vi "display_3s_stim_6s_ISI_12s_probes.vi"() -> ()   [LabVIEW 2019]
uses:
  <vilib>/Analysis/Matrix/Datatypes/RealMatrix.ctl
  <vilib>/Utility/file.llb/Write Delimited Spreadsheet (DBL).vi
  <vilib>/Analysis/Matrix/NI_Matrix.lvlib
panel:
  out "Num trials":u32=204
  out "ISI Time":dbl
  out "Stim TS":dbl
  out "Output":dbl[][](array[numeric])
  out "Output frame":T1
  out "Array temp1":T1
  out "Elapsed Time":dbl
  out "Display":bool=TRUE
  out "Trial":u32=1
  out "reward":dbl[](array[numeric])
  out "stim_id":dbl[](array[numeric])
  out "stim_loaded":dbl
  out "Timings":dbl[](array[numeric])
  out "Stimuli Loaded?":bool
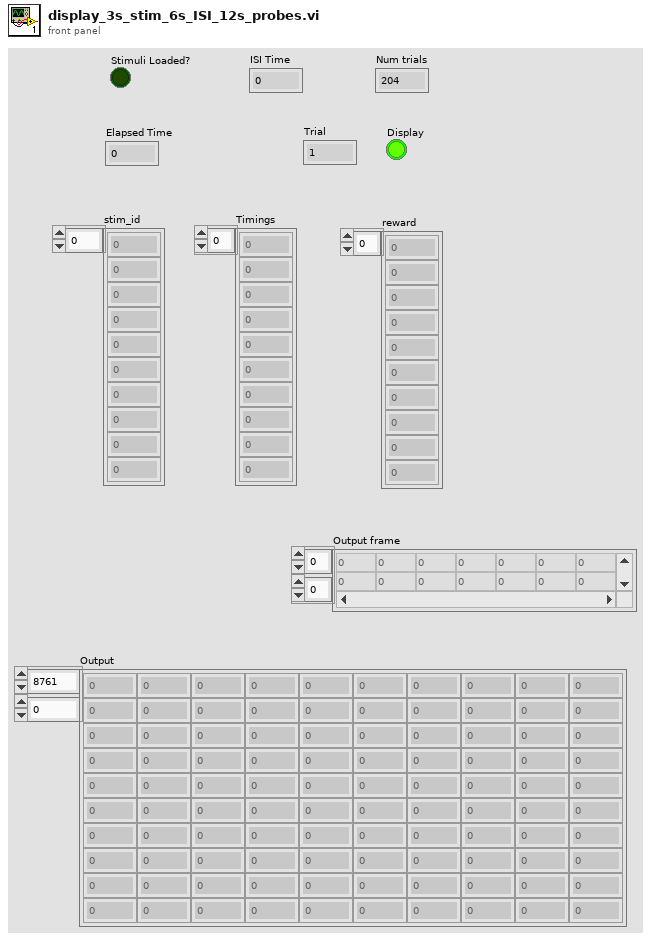
[diagram p1: front panel]
types:
  T1 = typedef "NI_Matrix.lvlib/RealMatrix.ctl" = dbl[][]
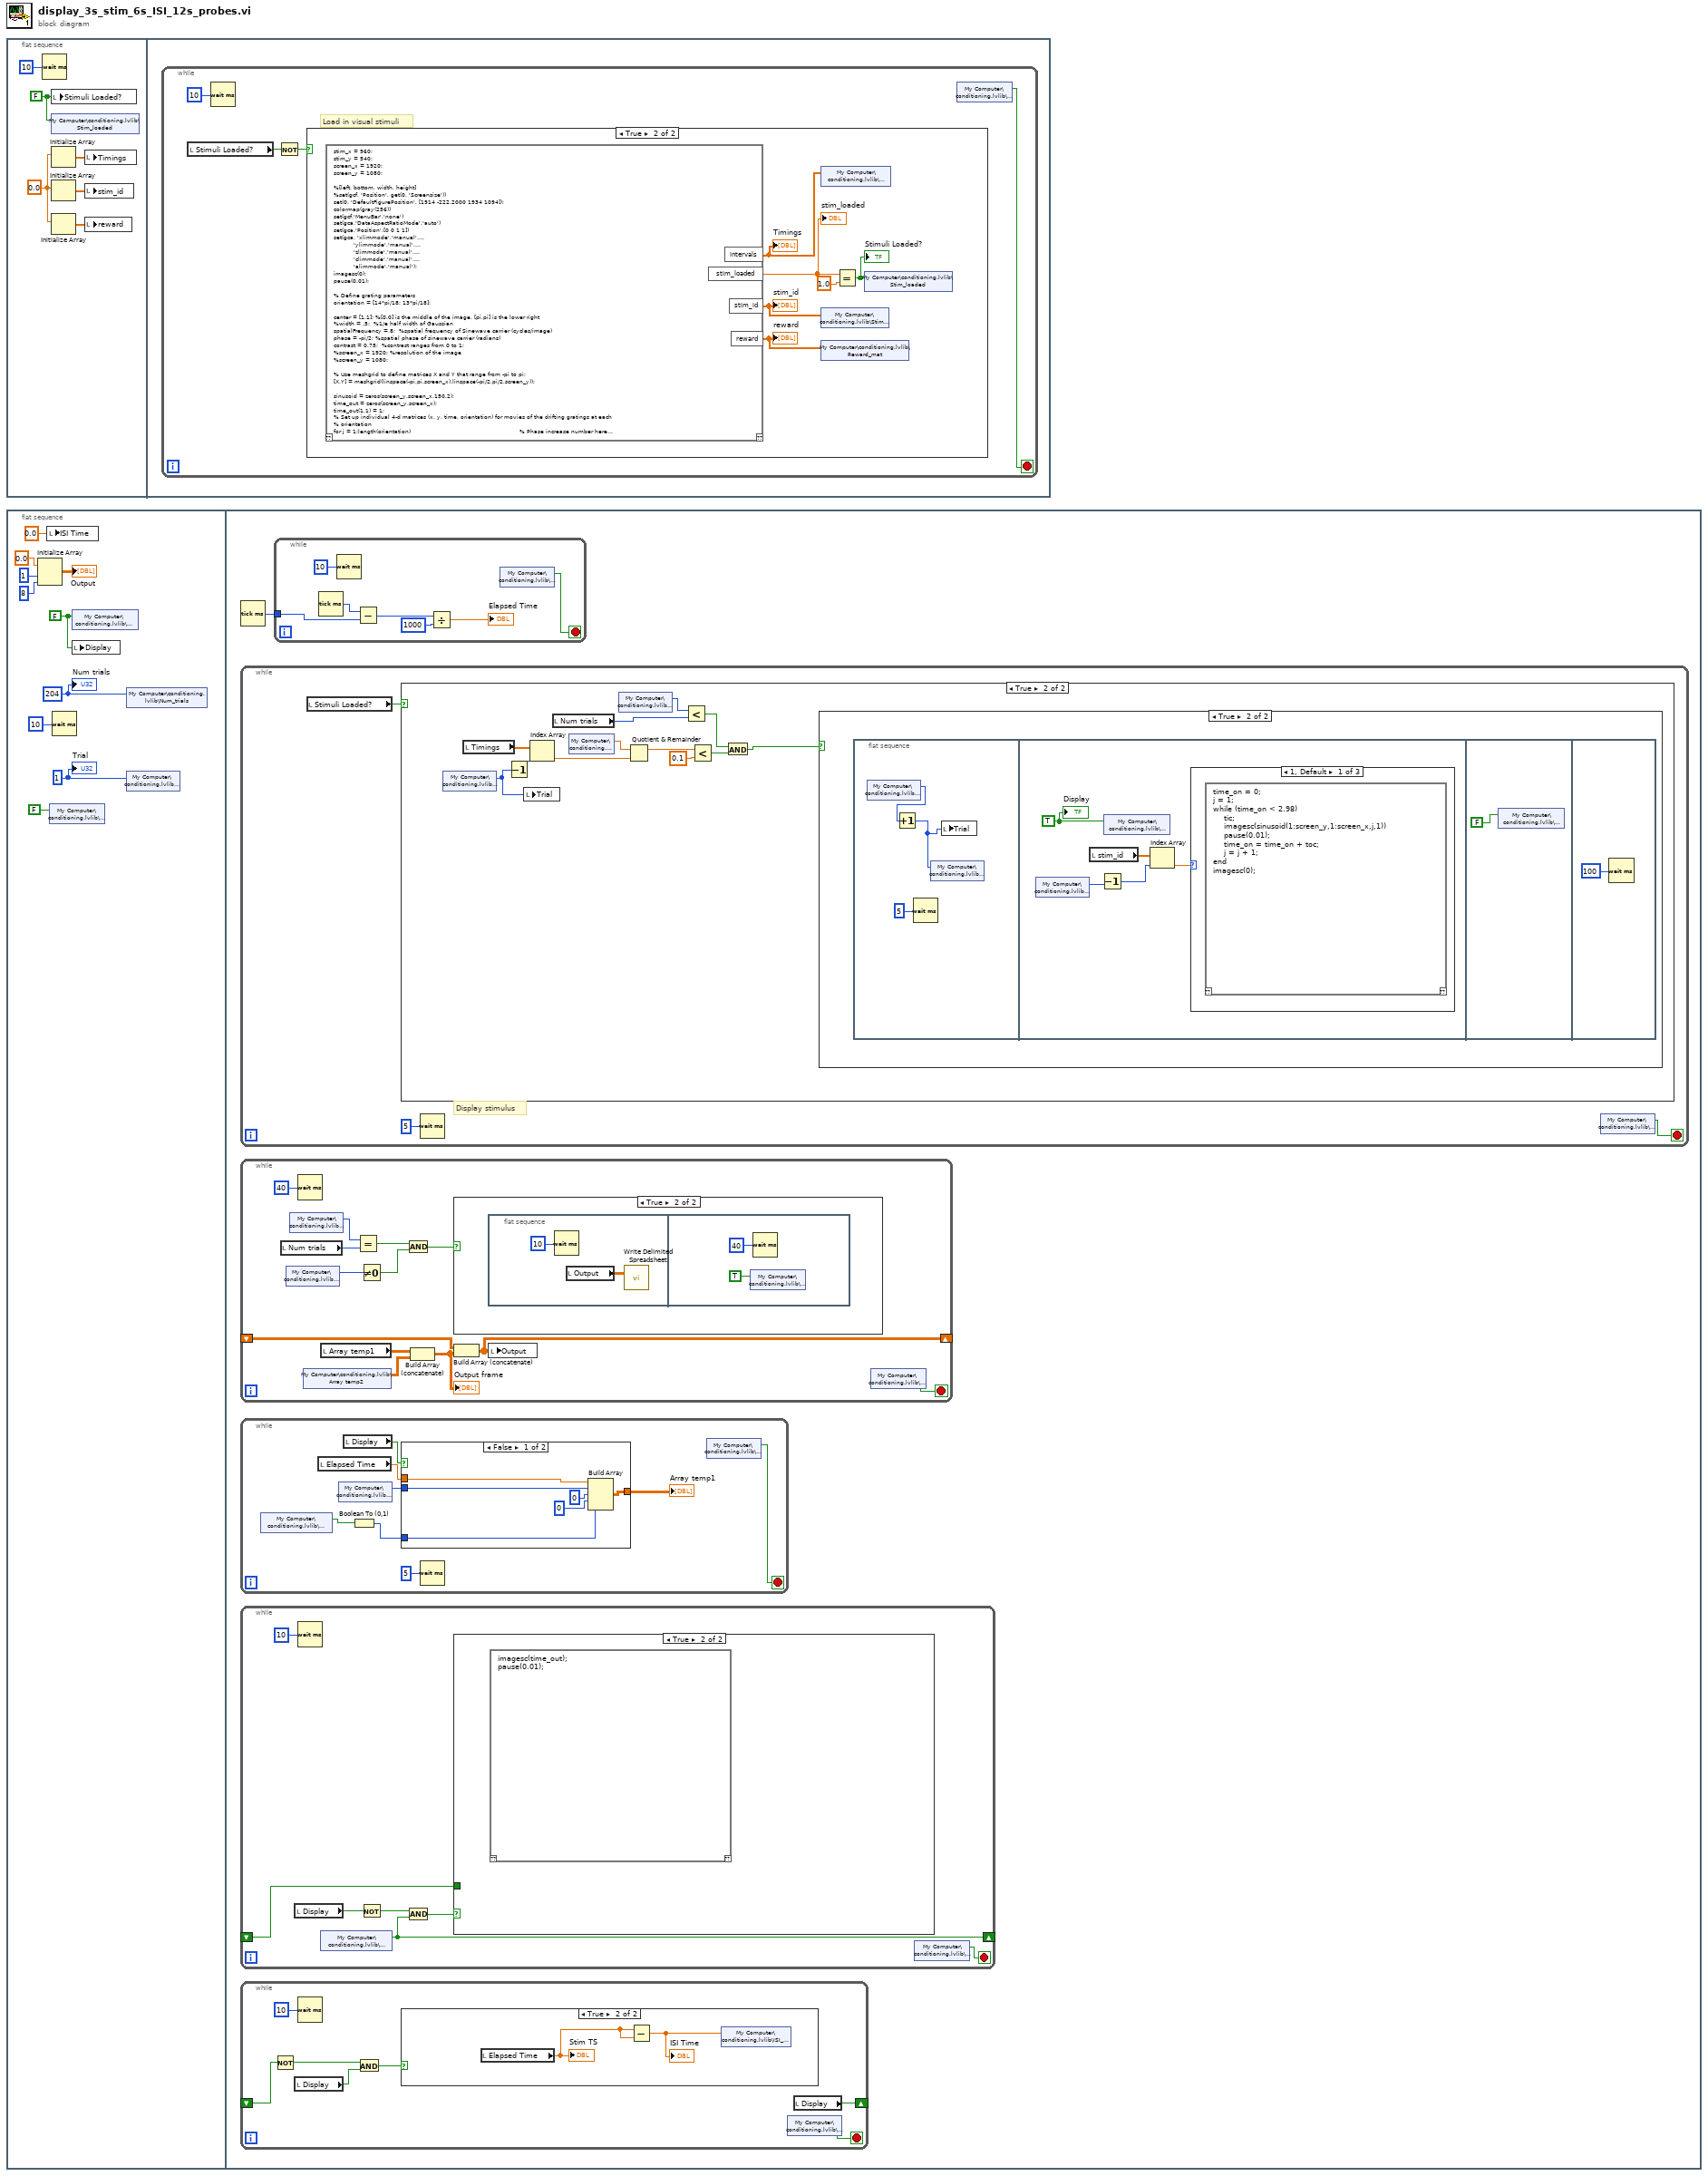
[diagram p0: block diagram]
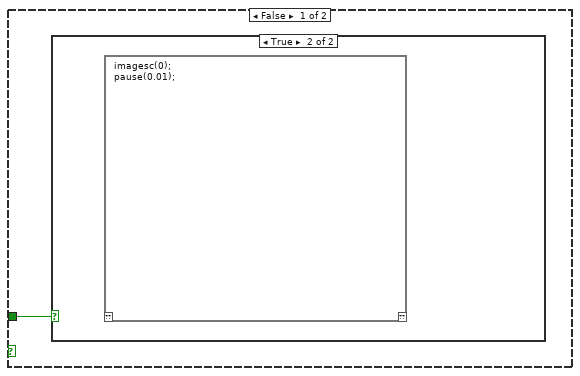
[diagram p3: hidden frame]
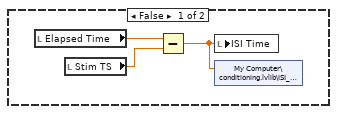
[diagram p5: hidden frame]
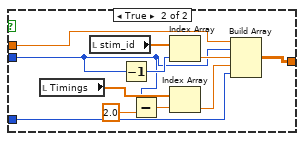
[diagram p6: hidden frame]
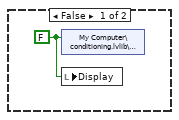
[diagram p9: hidden frame]
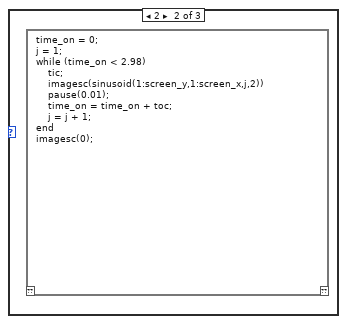
[diagram p10: hidden frame]
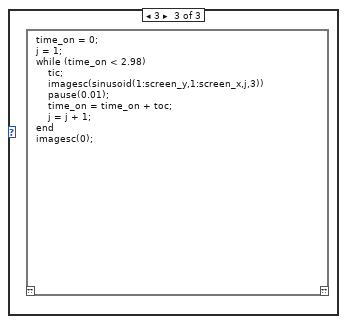
[diagram p11: hidden frame]
diagram:
  n1 = flat-sequence {
    frame #0 {
      w3 = 0.0 ("element")
      w1 = FALSE ("Stimuli Loaded?")
      n2 = Wait (ms)(milliseconds to wait=u32 10) -> ()  [unwired: 1 out]
      n3 = local write "Stimuli Loaded?"(w1) -> ()
      n4 = shared-variable "My Computer\\conditioning.lvlib\\Stim_loaded"(w1) -> ()  [unwired: 1 in, 1 out]
      n5 = Initialize Array(w3) -> (w5:dbl[])  [unwired: 1 in]
      n6 = Initialize Array(w3) -> (w4:dbl[])  [unwired: 1 in]
      n7 = Initialize Array(w3) -> (w2:dbl[])  [unwired: 1 in]
      n8 = local write "Timings"(w5) -> ()
      n9 = local write "stim_id"(w4) -> ()
      n10 = local write "reward"(w2) -> ()
    }
    frame #1 {
      n11 = while {
        stop <- w9 stop-if-true
        # "Load in visual stimuli"
        n12 = local read "Stimuli Loaded?"() -> (w8:bool)
        n13 = Wait (ms)(milliseconds to wait=u32 10) -> ()  [unwired: 1 out]
        n14 = Not(x=w8) -> (.not. x?=w7:bool)
        n15 = case shown="True" w7 {
          frame False {
          }
          frame True {
            n16 = script code="stim_x = 960;\nstim_y = 540;\nscreen_x = 1920;\nscreen_y = 1080;\n\n%[left, bottom, width, height]\n%set(gcf, 'Position', get(0, 'Screensize'))\nset(0, 'DefaultFigurePosition', [1914 -222.2000 1934 1094]);\ncolormap(gray(256))\nset(gcf,'MenuBar','none')\nset(gca,'DataAspectRatioMode','auto')\nset(gca,'Position',[0 0 1 1])\nset(gca, 'xlimmode','manual',...\n           'ylimmode','manual',...\n           'zlimmode','manual',...\n           'climmode','manual',...\n           'alimmode','manual');\nimagesc(0);\npause(0.01);\n\n% Define grating parameters\norientation = [14*pi/18; 13*pi/18];\n\ncenter = [1,1]; %[0,0] is the middle of the image, [pi,pi] is the lower right\n%width = .5;  %1/e half width of Gaussian\nspatialFrequency = 8;  %spatial frequency of Sinewave carrier (cycles/image)\nphase = -pi/2; %spatial phase of sinewave carrier (radians)\ncontrast = 0.75;  %contrast ranges from 0 to 1;\n%screen_x = 1920; %resolution of the image  \n%screen_y = 1080;\n\n% Use meshgrid to define matrices X and Y that range from -pi to pi;\n[X,Y] = meshgrid(linspace(-pi,pi,screen_x),linspace(-pi/2,pi/2,screen_y));\n\nsinusoid = zeros(screen_y,screen_x,150,2);\ntime_out = zeros(screen_y,screen_x);\ntime_out(1,1) = 1;\n% Set up individual 4-d matrices (x, y, time, orientation) for movies of the drifting gratings at each\n% orientation\nfor j = 1:length(orientation)                                                            % Phase increase number here\n    ramp(1:screen_y,1:screen_x,j) = cos(orientation(j))*(X-center(1)) + sin(orientation(j))*(Y-center(2));     %  |\n    for i = 1:150 %Sets the number of frames to define gratings for                   V\n       sinusoid(1:screen_y,1:screen_x,i,j) = contrast*sin(spatialFrequency*ramp(1:screen_y,1:screen_x,j)-...\n           (phase+(2*pi*(i-1)*(-30)/360))); %Number before '/360' sets the phase increase\n    end\nend\n\n%intervals = [ones(1,41)*10 ones(1,41)*11 ones(1,41)*12 ones(1,41)*13 ones(1,40)*14];\nintervals = [];\nfor i = 1:20\n   intervals = [intervals ones(1,9)*6 12];\nend\nintervals = [intervals 6 6 6 6];\n%intervals = [ones(1,204)*3];\nstim_id = [ones(1,204)*1];\n%reward = [ones(1,87)*1 ones(1,15)*0 ones(1,87)*1 ones(1,15)*0];\nreward = [ones(1,204)*1];\n\n%rand_idx1 = randperm(204);\n%rand_idx2 = randperm(204);\n%intervals = intervals(rand_idx2);\n%stim_id = stim_id(rand_idx2);\n%reward = reward(rand_idx2);\n\nstim_loaded = 1;" ("Script Node")() -> ("stim_loaded"=w16:dbl, "intervals"=w11:dbl[], "stim_id"=w12:dbl[], "reward"=w14:dbl[])  [unwired: 1 in, 1 out]
            "stim_loaded" <- w16
            "Timings" <- w11
            "stim_id" <- w12
            "reward" <- w14
            n17 = shared-variable "My Computer\\conditioning.lvlib\\Timings"(w11) -> ()  [unwired: 1 in, 1 out]
            n18 = shared-variable "My Computer\\conditioning.lvlib\\Stim_ID"(w12) -> ()  [unwired: 1 in, 1 out]
            n19 = shared-variable "My Computer\\conditioning.lvlib\\Reward_mat"(w14) -> ()  [unwired: 1 in, 1 out]
            n20 = Equal?(x=w16, y=1.0) -> (x = y?=w13:bool)
            "Stimuli Loaded?" <- w13
            n21 = shared-variable "My Computer\\conditioning.lvlib\\Stim_loaded"(w13) -> ()  [unwired: 1 in, 1 out]
          }
        }
        n22 = shared-variable "My Computer\\conditioning.lvlib\\Stop"() -> (w9:bool)  [unwired: 1 in, 1 out]
      }
    }
  }
  n23 = flat-sequence {
    frame #0 {
      w18 = u32 204
      w24 = FALSE ("Display")
      w26 = u32 1 ("Trial")
      n24 = Initialize Array(0.0 ("element"), 1 ("dimension size"), 8 ("dimension size")) -> (→"Output":dbl[][])
      n25 = local write "ISI Time"(0.0 ("ISI Time")) -> ()
      n26 = shared-variable "My Computer\\conditioning.lvlib\\Stop"(FALSE ("Stop")) -> ()  [unwired: 1 in, 1 out]
      n27 = Wait (ms)(milliseconds to wait=u32 10) -> ()  [unwired: 1 out]
      n28 = shared-variable "My Computer\\conditioning.lvlib\\Display"(w24) -> ()  [unwired: 1 in, 1 out]
      n29 = local write "Display"(w24) -> ()
      n30 = shared-variable "My Computer\\conditioning.lvlib\\Num_trials"(w18) -> ()  [unwired: 1 in, 1 out]
      n31 = shared-variable "My Computer\\conditioning.lvlib\\Trial"(w26) -> ()  [unwired: 1 in, 1 out]
      "Trial" <- w26
      "Num trials" <- w18
    }
    frame #1 {
      n32 = Tick Count (ms)() -> (millisecond timer value=w27:u32)
      n33 = while {
        stop <- w98 stop-if-true
        # "Display stimulus"
        n34 = local read "Stimuli Loaded?"() -> (w97:bool)
        n35 = case shown="True" w97 {
          frame False {
          }
          frame True {
            n36 = shared-variable "My Computer\\conditioning.lvlib\\Trial"() -> (w100:u32)  [unwired: 1 in, 1 out]
            n37 = local read "Timings"() -> (w109:dbl[])
            n38 = Decrement(x=w100) -> (x-1=w102:u32)
            n39 = local write "Trial"(w100) -> ()
            n40 = Index Array(array=w109, index=w102) -> (element=w108:dbl)
            n41 = local read "Num trials"() -> (w105:u32)
            n42 = shared-variable "My Computer\\conditioning.lvlib\\ISI"() -> (w104:dbl)  [unwired: 1 in, 1 out]
            n43 = shared-variable "My Computer\\conditioning.lvlib\\Trial"() -> (w101:u32)  [unwired: 1 in, 1 out]
            n44 = Quotient & Remainder(x=w104, y=w108) -> (x-y*floor(x/y)=w111:dbl)  [unwired: 1 out]
            n45 = Less?(x=w101, y=w105) -> (x < y?=w107:bool)
            n46 = Less?(x=w111, y=0.1) -> (x < y?=w106:bool)
            n47 = And(x=w107, y=w106) -> (x .and. y?=w103:bool)
            n48 = case shown="True" w103 {
              frame False {
                w112 = FALSE ("Display")
                n49 = shared-variable "My Computer\\conditioning.lvlib\\Display"(w112) -> ()  [unwired: 1 in, 1 out]
                n50 = local write "Display"(w112) -> ()
              }
              frame True {
                n51 = flat-sequence {
                  frame #0 {
                    n52 = shared-variable "My Computer\\conditioning.lvlib\\Trial"() -> (w114:u32)  [unwired: 1 in, 1 out]
                    n53 = Increment(x=w114) -> (x+1=w113:u32)
                    n54 = Wait (ms)(milliseconds to wait=u32 5) -> ()  [unwired: 1 out]
                    n55 = shared-variable "My Computer\\conditioning.lvlib\\Trial"(w113) -> ()  [unwired: 1 in, 1 out]
                    n56 = local write "Trial"(w113) -> ()
                  }
                  frame #1 {
                    w119 = TRUE ("Boolean")
                    n57 = shared-variable "My Computer\\conditioning.lvlib\\Trial"() -> (w116:u32)  [unwired: 1 in, 1 out]
                    n58 = local read "stim_id"() -> (w120:dbl[])
                    n59 = Decrement(x=w116) -> (x-1=w117:u32)
                    n60 = shared-variable "My Computer\\conditioning.lvlib\\Display"(w119) -> ()  [unwired: 1 in, 1 out]
                    n61 = Index Array(array=w120, index=w117) -> (element=w118:dbl)
                    n62 = case shown="1, Default" w118 {
                      frame 1, Default {
                        n63 = script code="time_on = 0;\nj = 1;\nwhile (time_on < 2.98)\n    tic;\n    imagesc(sinusoid(1:screen_y,1:screen_x,j,1))\n    pause(0.01);\n    time_on = time_on + toc;\n    j = j + 1;\nend\nimagesc(0);"() -> ()  [unwired: 1 in, 1 out]
                      }
                      frame 2 {
                        n64 = script code="time_on = 0;\nj = 1;\nwhile (time_on < 2.98)\n    tic;\n    imagesc(sinusoid(1:screen_y,1:screen_x,j,2))\n    pause(0.01);\n    time_on = time_on + toc;\n    j = j + 1;\nend\nimagesc(0);"() -> ()  [unwired: 1 in, 1 out]
                      }
                      frame 3 {
                        n65 = script code="time_on = 0;\nj = 1;\nwhile (time_on < 2.98)\n    tic;\n    imagesc(sinusoid(1:screen_y,1:screen_x,j,3))\n    pause(0.01);\n    time_on = time_on + toc;\n    j = j + 1;\nend\nimagesc(0);"() -> ()  [unwired: 1 in, 1 out]
                      }
                    }
                    "Display" <- w119
                  }
                  frame #2 {
                    n66 = shared-variable "My Computer\\conditioning.lvlib\\Display"(FALSE ("Display")) -> ()  [unwired: 1 in, 1 out]
                  }
                  frame #3 {
                    n67 = Wait (ms)(milliseconds to wait=u32 100) -> ()  [unwired: 1 out]
                  }
                }
              }
            }
          }
        }
        n68 = Wait (ms)(milliseconds to wait=u32 5) -> ()  [unwired: 1 out]
        n69 = shared-variable "My Computer\\conditioning.lvlib\\Stop"() -> (w98:bool)  [unwired: 1 in, 1 out]
      }
      n70 = while {
        shift-right: [w89] -> _
        shift-left: _ -> [w90]
        stop <- w92 stop-if-true
        n71 = local read "Num trials"() -> (w84:u32)
        n72 = shared-variable "My Computer\\conditioning.lvlib\\Trial"() -> (w80:u32)  [unwired: 1 in, 1 out]
        n73 = shared-variable "My Computer\\conditioning.lvlib\\Trial"() -> (w85:u32)  [unwired: 1 in, 1 out]
        n74 = Wait (ms)(milliseconds to wait=u32 40) -> ()  [unwired: 1 out]
        n75 = shared-variable "My Computer\\conditioning.lvlib\\Array temp2"() -> (w87:dbl[][])  [unwired: 1 in, 1 out]
        n76 = local read "Array temp1"() -> (w88:T1)
        n77 = Equal?(x=w85, y=w84) -> (x = y?=w83:bool)
        n78 = Not Equal To 0?(x=w80) -> (x != 0?=w82:bool)
        n79 = And(x=w83, y=w82) -> (x .and. y?=w81:bool)
        n80 = Build Array (concatenate)(w88, w87) -> (w86:T1)
        "Output frame" <- w86
        n81 = case shown="True" w81 {
          frame False {
          }
          frame True {
            n82 = flat-sequence {
              frame #0 {
                n83 = Wait (ms)(milliseconds to wait=u32 10) -> ()  [unwired: 1 out]
                n84 = local read "Output"() -> (w94:dbl[][])
                n85 = call-poly <vilib>:"Write Delimited Spreadsheet.vi"("2D data"=w94) -> ()  [unwired: 13 in, 2 out]
              }
              frame #1 {
                n86 = shared-variable "My Computer\\conditioning.lvlib\\Stop"(TRUE) -> ()  [unwired: 1 in, 1 out]
                n87 = Wait (ms)(milliseconds to wait=u32 40) -> ()  [unwired: 1 out]
              }
            }
          }
        }
        n88 = Build Array (concatenate) ("Build Matrix")(w90, w86) -> (w89:T1)
        n89 = local write "Output"(w89) -> ()
        n90 = shared-variable "My Computer\\conditioning.lvlib\\Stop"() -> (w92:bool)  [unwired: 1 in, 1 out]
      }
      n91 = while {
        stop <- w50 stop-if-true
        n92 = shared-variable "My Computer\\conditioning.lvlib\\Timeout"() -> (w49:bool)  [unwired: 1 in, 1 out]
        n93 = local read "Elapsed Time"() -> (w54:dbl)
        n94 = shared-variable "My Computer\\conditioning.lvlib\\Trial"() -> (w52:u32)  [unwired: 1 in, 1 out]
        n95 = local read "Display"() -> (w51:bool)
        n96 = Boolean To (0,1)(Boolean=w49) -> (0, 1=w48:i16)
        n97 = case shown="False" w51 {
          tunnel: w52 -> [w60 w63]
          tunnel: w54 -> [w61 w70]
          tunnel: [w59 w71] -> w53
          tunnel: w48 -> [w56 w65]
          frame False {
            n98 = Build Array(w61, w60, u32 0 ("milliseconds to wait"), 0, w56) -> (w59:T1)
          }
          frame True {
            n99 = local read "Timings"() -> (w68:dbl[])
            n100 = local read "stim_id"() -> (w72:dbl[])
            n101 = Decrement(x=w63) -> (x-1=w67:u32)
            n102 = Subtract(x=w63, y=2.0) -> (x-y=w62:dbl)
            n103 = Index Array(array=w72, index=w67) -> (element=w69:dbl)
            n104 = Index Array(array=w68, index=w62) -> (element=w66:dbl)
            n105 = Build Array(w70, w63, w69, w66, w65) -> (w71:T1)
          }
        }
        "Array temp1" <- w53
        n106 = Wait (ms)(milliseconds to wait=u32 5) -> ()  [unwired: 1 out]
        n107 = shared-variable "My Computer\\conditioning.lvlib\\Stop"() -> (w50:bool)  [unwired: 1 in, 1 out]
      }
      n108 = while {
        shift-right: [w29] -> _
        shift-left: _ -> [w28]
        stop <- w34 stop-if-true
        n109 = local read "Display"() -> (w31:bool)
        n110 = Wait (ms)(milliseconds to wait=u32 10) -> ()  [unwired: 1 out]
        n111 = shared-variable "My Computer\\conditioning.lvlib\\Timeout"() -> (w29:bool)  [unwired: 1 in, 1 out]
        n112 = Not(x=w31) -> (.not. x?=w32:bool)
        n113 = And(x=w32, y=w29) -> (x .and. y?=w30:bool)
        n114 = case shown="True" w30 {
          tunnel: w28 -> [w35 _]
          frame False {
            n115 = case shown="True" w35 {
              frame False {
              }
              frame True {
                n116 = script code="imagesc(0);\npause(0.01);"() -> ()  [unwired: 1 in, 1 out]
              }
            }
          }
          frame True {
            n117 = script code="imagesc(time_out);\npause(0.01);"() -> ()  [unwired: 1 in, 1 out]
          }
        }
        n118 = shared-variable "My Computer\\conditioning.lvlib\\Stop"() -> (w34:bool)  [unwired: 1 in, 1 out]
      }
      n119 = while {
        shift-right: [w40] -> _
        shift-left: _ -> [w39]
        stop <- w42 stop-if-true
        n120 = Not(x=w39) -> (.not. x?=w38:bool)
        n121 = local read "Display"() -> (w37:bool)
        n122 = Wait (ms)(milliseconds to wait=u32 10) -> ()  [unwired: 1 out]
        n123 = And(x=w38, y=w37) -> (x .and. y?=w36:bool)
        n124 = case shown="True" w36 {
          frame False {
            n125 = local read "Elapsed Time"() -> (w43:dbl)
            n126 = local read "Stim TS"() -> (w45:dbl)
            n127 = Subtract(x=w43, y=w45) -> (x-y=w44:dbl)
            n128 = local write "ISI Time"(w44) -> ()
            n129 = shared-variable "My Computer\\conditioning.lvlib\\ISI_Time"(w44) -> ()  [unwired: 1 in, 1 out]
          }
          frame True {
            n130 = local read "Elapsed Time"() -> (w46:dbl)
            "Stim TS" <- w46
            n131 = Subtract(x=w46, y=w46) -> (x-y=w47:dbl)
            "ISI Time" <- w47
            n132 = shared-variable "My Computer\\conditioning.lvlib\\ISI_Time"(w47) -> ()  [unwired: 1 in, 1 out]
          }
        }
        n133 = shared-variable "My Computer\\conditioning.lvlib\\Stop"() -> (w42:bool)  [unwired: 1 in, 1 out]
        n134 = local read "Display"() -> (w40:bool)
      }
      n135 = while {
        tunnel: w27 -> [w76]
        stop <- w73 stop-if-true
        n136 = Tick Count (ms)() -> (millisecond timer value=w77:u32)
        n137 = Wait (ms)(milliseconds to wait=u32 10) -> ()  [unwired: 1 out]
        n138 = Subtract(x=w77, y=w76) -> (x-y=w74:u32)
        n139 = Divide(x=w74, y=u32 1000) -> (x/y=→"Elapsed Time":dbl)
        n140 = shared-variable "My Computer\\conditioning.lvlib\\Stop"() -> (w73:bool)  [unwired: 1 in, 1 out]
      }
    }
  }
